vi "Exit.vi"   [LabVIEW 2015]
uses:
  Global/Globalclient.vi
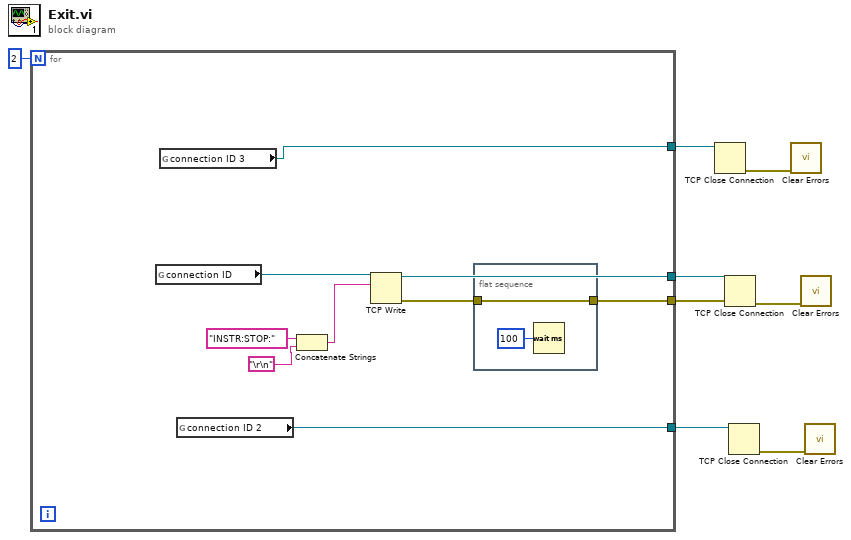
[diagram p0: block diagram]
diagram:
  n1 = for {
    N: 2 -> [_]
    tunnel: [w15] -> w7
    tunnel: [w14] -> w6
    tunnel: [w10] -> w3
    tunnel: [w9] -> w1
    n2 = global read "Globalclient.vi" "connection ID"() -> (w16:refnum<k5>)
    n3 = global read "Globalclient.vi" "connection ID 3"() -> (w9:refnum<k5>)
    n4 = global read "Globalclient.vi" "connection ID 2"() -> (w10:refnum<k5>)
    n5 = Concatenate Strings("INSTR:STOP:" ("string"), "\r\n") -> (w11:string)
    n6 = TCP Write(connection ID=w16, data in=w11) -> (connection ID out=w14:refnum<k5>, error out=w17:errorcluster)  [unwired: 2 in, 1 out]
    n7 = flat-sequence {
      tunnel: w17 -> [w18]
      tunnel: [w18] -> w15
      frame #0 {
        n8 = Wait (ms)(milliseconds to wait=u32 100 ("等待时间（毫秒）")) -> ()  [unwired: 1 out]
      }
    }
  }
  n9 = TCP Close Connection(connection ID=w1) -> (error out=w2:errorcluster)  [unwired: 2 in, 1 out]
  n10 = TCP Close Connection(connection ID=w6, error in (no error)=w7) -> (error out=w5:errorcluster)  [unwired: 1 in, 1 out]
  n11 = TCP Close Connection(connection ID=w3) -> (error out=w4:errorcluster)  [unwired: 2 in, 1 out]
  n12 = call <vilib>:"Clear Errors.vi"("error in (no error)"=w2) -> ()  [unwired: 5 in, 2 out]
  n13 = call <vilib>:"Clear Errors.vi"("error in (no error)"=w5) -> ()  [unwired: 5 in, 2 out]
  n14 = call <vilib>:"Clear Errors.vi"("error in (no error)"=w4) -> ()  [unwired: 5 in, 2 out]
